vi "create standard response header.vi"() -> (3 "default header":T1)   [LabVIEW 2016, in "http responder.lvclass"]
uses:
  http responder.lvclass
  HTTP server/http header data.ctl
  HTTP server/Basic HTTP server.lvclass
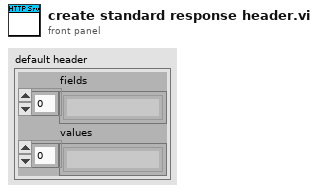
[diagram p1: front panel]
types:
  T1 = typedef "Basic HTTP server.lvclass/http header data.ctl" = cluster{"fields":string[], "values":string[]}
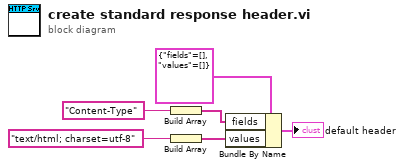
[diagram p0: block diagram]
diagram:
  n1 = Build Array("Content-Type" ("name")) -> (w5:string[])
  n2 = Build Array("text/html; charset=utf-8" ("name")) -> (w3:string[])
  n3 = Bundle By Name(cluster=T1 {"fields"=[], "values"=[]} ("headers"), "fields"=w5, "values"=w3) -> (→"default header":T1)
